vi "keccak.fpga.step.8.vi"(11 "Exy.in":u64[](array[numeric])=[0, 0, 0, 0, 0, 0, 0, 0, 0, 0, 0, 0, 0, 0, 0, 0, 0, 0, 0, 0, 0, 0, 0, 0, 0]) -> (3 "Step.8.Dx":u64[](array[numeric]))   [LabVIEW 2021]
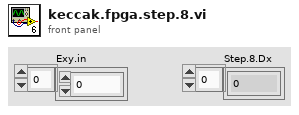
[diagram p1: front panel]
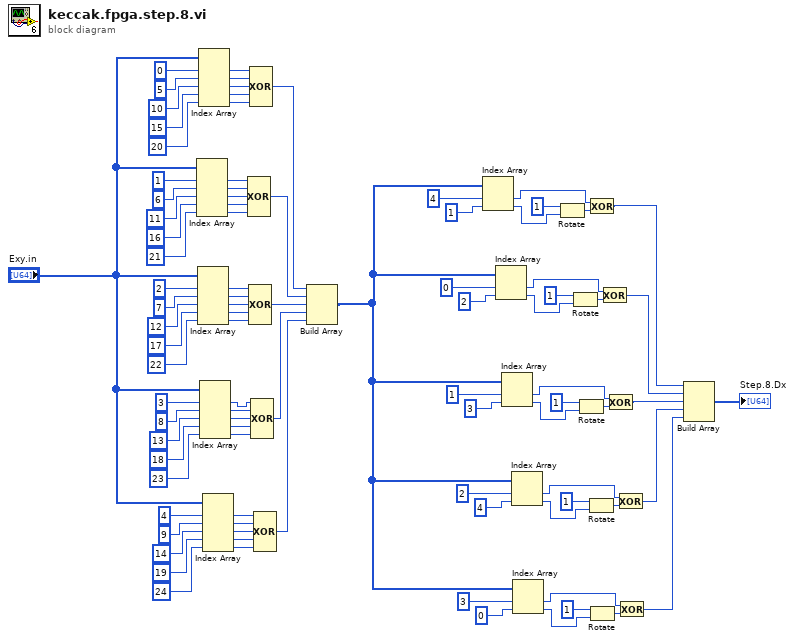
[diagram p0: block diagram]
diagram:
  n1 = Index Array(array="Exy.in", index #1=1 ("index (row)"), index #2=6 ("index"), index #3=11 ("index"), index #4=16 ("index"), index #5=21 ("index")) -> (element #1=w38:u64, element #2=w78:u64, element #3=w77:u64, element #4=w76:u64, element #5=w75:u64)
  n2 = Index Array(array="Exy.in", index #1=2 ("index (row)"), index #2=7 ("index"), index #3=12 ("index"), index #4=17 ("index"), index #5=22 ("index")) -> (element #1=w43:u64, element #2=w70:u64, element #3=w69:u64, element #4=w68:u64, element #5=w67:u64)
  n3 = Index Array(array="Exy.in", index #1=0 ("index (row)"), index #2=5 ("index"), index #3=10 ("index"), index #4=15 ("index"), index #5=20 ("index")) -> (element #1=w88:u64, element #2=w87:u64, element #3=w86:u64, element #4=w85:u64, element #5=w84:u64)
  n4 = Index Array(array="Exy.in", index #1=3 ("index (row)"), index #2=8 ("index"), index #3=13 ("index"), index #4=18 ("index"), index #5=23 ("index")) -> (element #1=w44:u64, element #2=w62:u64, element #3=w61:u64, element #4=w60:u64, element #5=w59:u64)
  n5 = Index Array(array="Exy.in", index #1=4 ("index (row)"), index #2=9 ("index"), index #3=14 ("index"), index #4=19 ("index"), index #5=24 ("index")) -> (element #1=w45:u64, element #2=w54:u64, element #3=w53:u64, element #4=w52:u64, element #5=w51:u64)
  n6 = Compound Arithmetic op=XOR(w38, w78, w77, w76, w75) -> (w46:u64)
  n7 = Compound Arithmetic op=XOR(w43, w70, w69, w68, w67) -> (w47:u64)
  n8 = Compound Arithmetic op=XOR(w88, w87, w86, w85, w84) -> (w83:u64)
  n9 = Compound Arithmetic op=XOR(w44, w62, w61, w60, w59) -> (w48:u64)
  n10 = Compound Arithmetic op=XOR(w45, w54, w53, w52, w51) -> (w49:u64)
  n11 = Build Array(w83, w46, w47, w48, w49) -> (w4:u64[])
  n12 = Index Array(array=w4, index #1=4 ("index"), index #2=1 ("index")) -> (element #1=w35:u64, element #2=w33:u64)
  n13 = Index Array(array=w4, index #1=0 ("index"), index #2=2 ("index")) -> (element #1=w28:u64, element #2=w26:u64)
  n14 = Index Array(array=w4, index #1=1 ("index"), index #2=3 ("index")) -> (element #1=w22:u64, element #2=w20:u64)
  n15 = Index Array(array=w4, index #1=2 ("index"), index #2=4 ("index")) -> (element #1=w16:u64, element #2=w14:u64)
  n16 = Index Array(array=w4, index #1=3 ("index"), index #2=0 ("index")) -> (element #1=w10:u64, element #2=w8:u64)
  n17 = Rotate(1:w33, 2:i16 1 ("y")) -> (0:w34:u64)
  n18 = Rotate(1:w26, 2:i16 1 ("y")) -> (0:w27:u64)
  n19 = Rotate(1:w20, 2:i16 1 ("y")) -> (0:w21:u64)
  n20 = Rotate(1:w14, 2:i16 1 ("y")) -> (0:w15:u64)
  n21 = Exclusive Or(1:w34, 2:w35) -> (0:w32:u64)
  n22 = Rotate(1:w8, 2:i16 1 ("y")) -> (0:w9:u64)
  n23 = Exclusive Or(1:w27, 2:w28) -> (0:w5:u64)
  n24 = Exclusive Or(1:w21, 2:w22) -> (0:w3:u64)
  n25 = Exclusive Or(1:w15, 2:w16) -> (0:w2:u64)
  n26 = Exclusive Or(1:w9, 2:w10) -> (0:w1:u64)
  n27 = Build Array(w32, w5, w3, w2, w1) -> (→"Step.8.Dx":u64[])
